vi "to table.vi"(8 "error in":errorcluster, 10 "variant":variant, 11 "shared memory module configuration":refnum<class "Shared Memory Configuration.lvclass">) -> (0 "error out":errorcluster, 2 "table":string[][](array[string]), 3 "shared memory module configuration out":refnum<class "Shared Memory Configuration.lvclass">)   [LabVIEW 2013, in "Shared Memory Configuration.lvclass"]
doc: "Copyright 2016 National Instruments Corporation\n\nLicensed under the Apache License, Version 2.0 (the \"License\"); you may not use this file except in compliance with the License. You may obtain a copy of the License at http://www.apache.org/licenses/LICENSE-2.0\nUnless required by applicable law or agreed to in writing, software distributed under the License is distributed on an \"AS IS\" BASIS, WITHOUT WARRANTIES OR CONDITIONS OF ANY KIND, either express or implied. See the License for the specific language governing permissions and limitations under the License."
uses:
  Shared Memory Configuration.lvclass
  <vilib>/NI/Module Execution Interface/Engine Configuration/engine configuration.lvclass
  Shared Memory Configuration.lvclass/Shared Memory Configuration.ctl
  <vilib>/NI/Configuration Framework/serializable configuration/NISE_CEF_serializable configuration.lvclass/NISE_CEF_serializable configuration.ctl
  <vilib>/NI/Tag Bus/tag/tag descriptor.lvclass/tag descriptor.ctl
  Read lines.vi
  <vilib>/Utility/LVClass/Get LV Class Name.vi
  <vilib>/NI/Configuration Framework/error generator/NISE_error generator.vi
  <vilib>/NI/Tag Bus/tag/tag descriptor.lvclass
  <vilib>/NI/Configuration Framework/serializable configuration/NISE_CEF_serializable configuration.lvclass
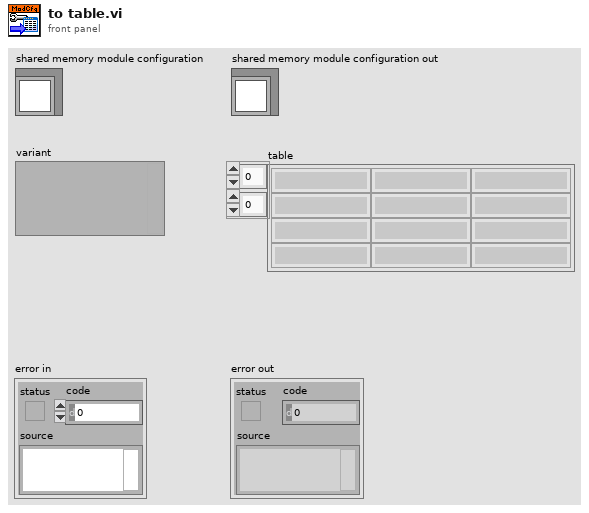
[diagram p1: front panel]
types:
  T1 = typedef "Shared Memory Configuration.lvclass/line configuration.ctl" = cluster{"name":string, "data type":T2, "channel":refnum<class "TBM channel.lvclass">}
  T2 = typedef "tag bus.lvlib/tag descriptor.lvclass/Data Type.ctl" = enum16{"Double", "Single", "I64", "I32", "I16", "I8", "U64", "U32", "U16", "U8", "Boolean", "String", "Array of Double", "Array of Single", "Array of I64", "Array of I32", "Array of I16", "Array of I8", "Array of U64", "Array of U32", "Array of U16", "Array of U8", "Array of Boolean", "Array of String"}
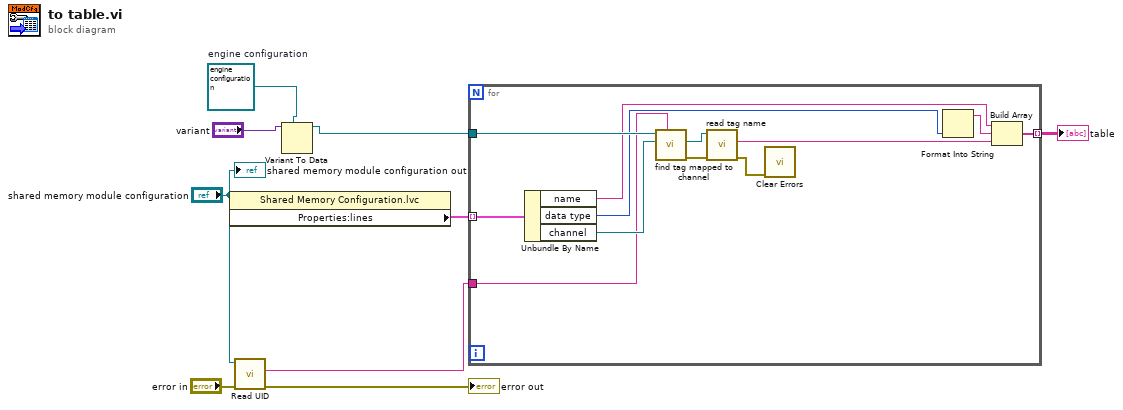
[diagram p0: block diagram]
diagram:
  w1 = refnum<class "engine configuration.lvclass"> refnum  # engine configuration
  n1 = property class="Shared Memory Configuration.lvc"(reference="shared memory module configuration") -> ("Properties:lines"=w8:T1[])  [unwired: 1 in, 2 out]
  n2 = call <vilib>:"Read UID.vi"("error in"="error in", "configuration in"="shared memory module configuration") -> ("error out"=→"error out":errorcluster, "instance id"=w9:string)  [unwired: 7 in, 1 out]
  n3 = Variant To Data(type=w1, Variant="variant") -> (data=w3:refnum<class "engine configuration.lvclass">)  [unwired: 1 in, 1 out]
  n4 = for {
    tunnel: w8 -> [w21] mode=indexing
    tunnel: w3 -> [w20]
    tunnel: w9 -> [w10]
    tunnel: [w13] -> w7 mode=indexing
    n5 = Unbundle By Name(w21) -> ("name"=w16:string, "data type"=w15:T2, "channel"=w18:refnum<class "TBM channel.lvclass">)
    n6 = call <vilib>:"find tag mapped to channel.vi"("owner"=w10, "channel"=w18, "engine configuration in"=w20) -> ("error out"=w12:errorcluster, "tag"=w19:refnum<class "tag descriptor.lvclass">)  [unwired: 6 in, 1 out]
    n7 = call <vilib>:"read tag name.vi"("error in"=w12, "system tag in"=w19) -> ("error out"=w11:errorcluster, "name"=w17:string)  [unwired: 7 in, 1 out]
    n8 = call <vilib>:"Clear Errors.vi"("error in (no error)"=w11) -> ()  [unwired: 6 in, 1 out]
    n9 = Format Into String(w15) -> (resulting string=w14:string)  [unwired: 3 in, 1 out]
    n10 = Build Array(w16, w14, w17) -> (w13:string[])
  }
  "table" <- w7
  "shared memory module configuration out" <- "shared memory module configuration"
